vi "MQTT_Publicar_Mensaje.vi"() -> ()   [LabVIEW 2017, in "MQTT_Functions.lvlib"]
doc: "A simple client example that connects to a broker server and publishes messages to a topic.\n\n© 2015 - daq.io, LLC - Peter Adelhardt"
uses:
  MQTT_Functions.lvlib
  Controls/QoS.ctl
  Controls/Retain_Flag.ctl
  Controls/DUP_Flag.ctl
  Controls/Connection_Return_Codes.ctl
  Controls/Connect_Flags.ctl
panel:
  out "Message published":string
  in  "Stop Publishing":bool
  out "Message ID (acknowledged)":u16=10
  out "Acknowledged":bool
  in  "Message ID":u16=20
  in  "MQTT Broker":cluster{"address (IP)":string, "port":u16}={"address (IP)"="broker.hivemq.com", "port"=1883}
  in  "Message to be published":string="LabVIEW says it's "
  out "Connection Status":T1=enum."Connection refused: not authorized"
  out "error out":errorcluster
  in  "Client ID":string="LabVIEW_MQTT_Client"
  in  "error in (no error)":errorcluster
  in  "Topic":string="testtopic/LVMQTT"
  in  "Publish Meta":cluster{"QoS":T2, "Retain":T3, "DUP":T4}
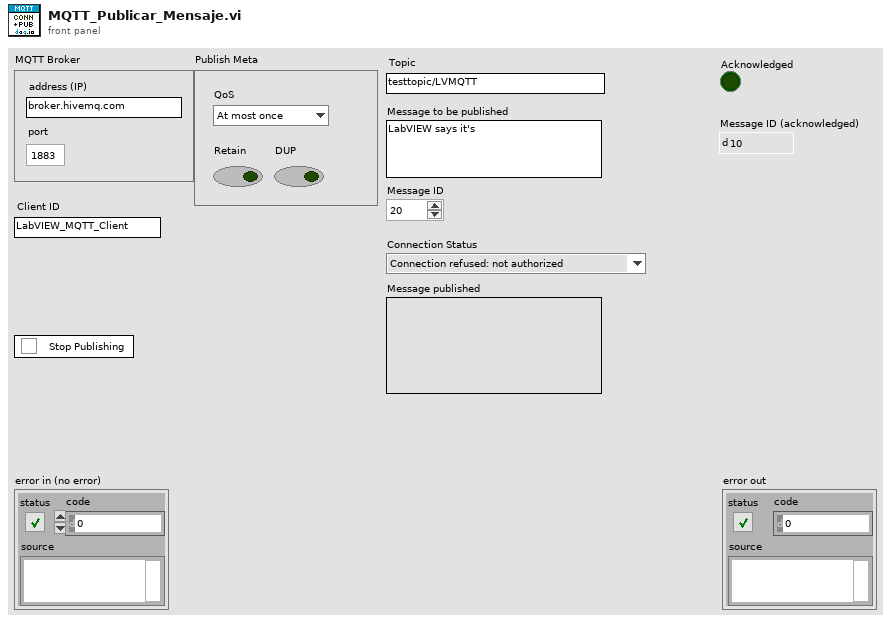
[diagram p1: front panel]
types:
  T1 = typedef "MQTT_Functions.lvlib/Connection_Return_Codes.ctl" = enum16{"Connection accepted", "Connection refused: unacceptable protocol version", "Connection refused: identifier rejected", "Connection refused: Server unavailable", "Connection refused: bad user name or password", "Connection refused: not authorized"}
  T2 = typedef "MQTT_Functions.lvlib/QoS.ctl" = enum8{"At most once", "At least once", "Exactly once", "Reserved"}
  T3 = typedef "MQTT_Functions.lvlib/Retain_Flag.ctl" = bool
  T4 = typedef "MQTT_Functions.lvlib/DUP_Flag.ctl" = bool
  T5 = typedef "MQTT_Functions.lvlib/Connect_Flags.ctl" = cluster{"user name":bool, "password":bool, "will retain":bool, "will flag":bool, "clean session":bool, "reserved":bool, "will QoS":T2}
  T6 = cluster{"QoS":T2, "DUP":T4, "Retain":T3, "Keep Alive (sec)":u16}
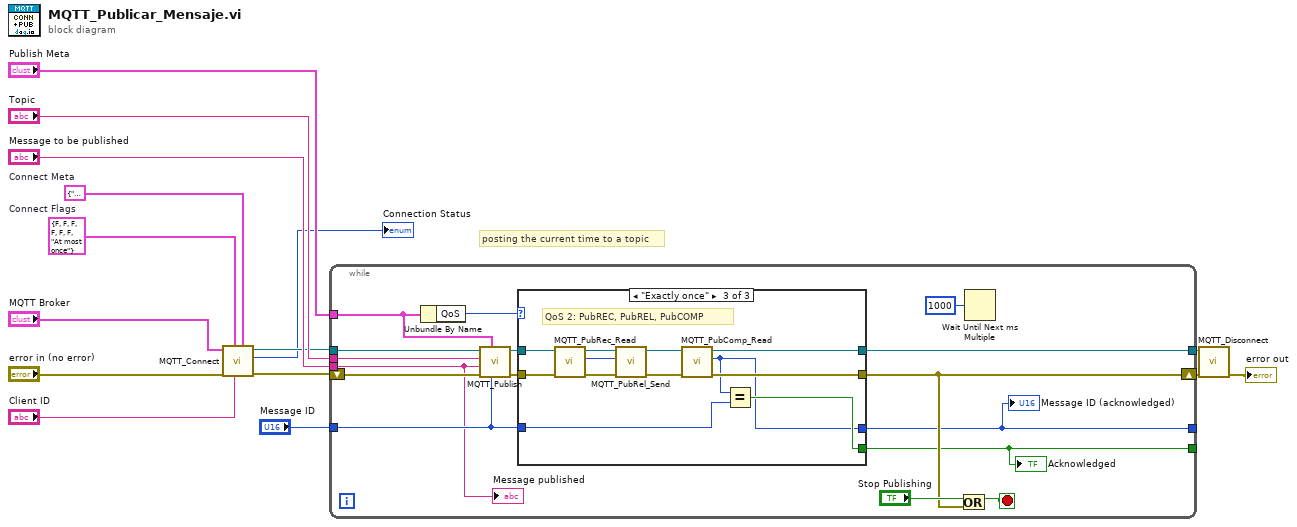
[diagram p0: block diagram]
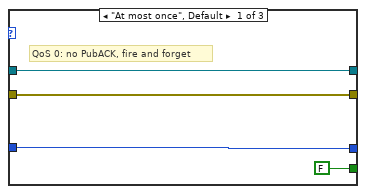
[diagram p2: hidden frame]
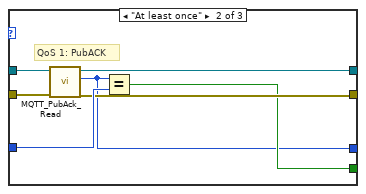
[diagram p3: hidden frame]
diagram:
  w13 = T5 {"user name"=FALSE, "password"=FALSE, "will retain"=FALSE, "will flag"=FALSE, "clean session"=FALSE, "reserved"=FALSE, "will QoS"=enum."At most once"}  # Connect Flags
  w10 = T6 {"QoS"=enum."At most once", "DUP"=FALSE, "Retain"=FALSE, "Keep Alive (sec)"=60}  # Connect Meta
  # "posting the current time to a topic"
  n1 = call "MQTT_Connect.vi"("Connect Meta"=w10, "Client ID"="Client ID", "Connect Flags"=w13, "error in (no error)"="error in (no error)", "MQTT Broker"="MQTT Broker") -> ("error out"=w1:errorcluster, "Connection Status"=→"Connection Status":T1, "connection ID out"=w3:refnum<k5>)  [unwired: 4 in]
  n2 = while {
    tunnel: "Topic" -> [w31]
    tunnel: "Message to be published" -> [w16]
    tunnel: w3 -> [w30]
    tunnel: "Publish Meta" -> [w28]
    tunnel: [w24] -> w6
    tunnel: "Message ID" -> [w23]
    tunnel: [w18] -> _
    tunnel: [w17] -> _
    shift-right: [w20] -> w7
    shift-left: w1 -> [w29]
    stop <- w21 stop-if-true
    n3 = Unbundle By Name(w28) -> ("QoS"=w27:T2)
    n4 = call "MQTT_Publish.vi"("Message ID"=w23, "Publish Meta"=w28, "error in (no error)"=w29, "Message to be published"=w16, "Topic"=w31, "connection ID"=w30) -> ("error out"=w26:errorcluster, "connection ID out"=w25:refnum<k5>)  [unwired: 4 in]
    n5 = case shown="\"Exactly once\"" w27 {
      tunnel: w26 -> [w34 w41 w53]
      tunnel: w25 -> [w35 w42 w54]
      tunnel: [w34 w39 w46] -> w20
      tunnel: [w35 w38 w47] -> w24
      tunnel: w23 -> [w32 w40 w52]
      tunnel: [FALSE w37 w48] -> w18
      tunnel: [w32 w36 w45] -> w17
      frame "At most once", Default {
        # "QoS 0: no PubACK, fire and forget"
      }
      frame "At least once" {
        # "QoS 1: PubACK"
        n6 = call "MQTT_PubAck_Read.vi"("error in (no error)"=w41, "connection ID"=w42) -> ("error out"=w39:errorcluster, "Message ID"=w36:u16, "connection ID out"=w38:refnum<k5>)  [unwired: 7 in]
        n7 = Equal?(x=w36, y=w40) -> (x = y?=w37:bool)
      }
      frame "Exactly once" {
        # "QoS 2: PubREC, PubREL, PubCOMP"
        n8 = call "MQTT_PubRec_Read.vi"("error in (no error)"=w53, "connection ID"=w54) -> ("error out"=w51:errorcluster, "Message ID"=w49:u16, "connection ID out"=w50:refnum<k5>)  [unwired: 7 in]
        n9 = call "MQTT_PubRel_Send.vi"("error in (no error)"=w51, "Message ID"=w49, "connection ID"=w50) -> ("error out"=w43:errorcluster, "connection ID out"=w44:refnum<k5>)  [unwired: 6 in, 1 out]
        n10 = call "MQTT_PubComp_Read.vi"("error in (no error)"=w43, "connection ID"=w44) -> ("error out"=w46:errorcluster, "Message ID"=w45:u16, "connection ID out"=w47:refnum<k5>)  [unwired: 7 in]
        n11 = Equal?(x=w45, y=w52) -> (x = y?=w48:bool)
      }
    }
    "Message ID (acknowledged)" <- w17
    "Acknowledged" <- w18
    n12 = Or(x="Stop Publishing", y=w20) -> (x .or. y?=w21:bool)
    n13 = Wait Until Next ms Multiple(millisecond multiple=u32 1000) -> ()  [unwired: 1 out]
    "Message published" <- w16
  }
  n14 = call "MQTT_Disconnect.vi"("error in (no error)"=w7, "connection ID"=w6) -> ("error out"=→"error out":errorcluster)  [unwired: 9 in]
